vi "DiffDriveSim_FindEncoder.vi"(9 "Restart":bool, 10 "Enc B DI Channel":T1, 11 "Enc A DI Channel":T1) -> (1 "Found":bool, 3 "EncoderIndex":T2)   [LabVIEW 2019]
uses:
  <vilib>/Rock Robotics/SystemInterfaces/Encoder/FPGA_EncoderIdx.ctl
  <vilib>/Rock Robotics/SystemInterfaces/DIO/FPGA_DIOChannel.ctl
  <vilib>/Rock Robotics/WPI/Simulation/Protocol/Devices/Encoder/Encoder Update Ops.ctl
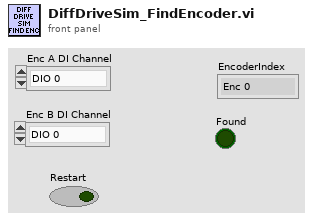
[diagram p1: front panel]
types:
  T1 = typedef "FPGA_DIOChannel.ctl" = enum8{"DIO 0", "DIO 1", "DIO 2", "DIO 3", "DIO 4", "DIO 5", "DIO 6", "DIO 7", "DIO 8", "DIO 9", "DIO MXP 0", "DIO MXP 1", "DIO MXP 2", "DIO MXP 3", "DIO MXP 4", "DIO MXP 5", "DIO MXP 6", "DIO MXP 7", "DIO MXP 8", "DIO MXP 9", "DIO MXP 10", "DIO MXP 11", "DIO MXP 12", "DIO MXP 13", "DIO MXP 14", "DIO MXP 15", "SPI Port CS1", "SPI Port CS2", "SPI Port CS3", "SPI Port MISO", "SPI Port MOSI", "Invalid"}
  T2 = typedef "FPGA_EncoderIdx.ctl" = enum8{"Enc 0", "Enc 1", "Enc 2", "Enc 3", "Enc 4", "Enc 5", "Enc 6", "Enc 7", "Invalid"}
  T3 = typedef "Encoder Update Ops.ctl" = enum16{"set init", "set count", "set period", "set reset", "set samples_to_avg", "get", "delete", "JSON update", "set name", "transmit initial", "reset", "set channel_a", "set channel_b", "set values"}
  T4 = typedef "Encoder proto.ctl" = cluster{"type":string, "device":string, "name":string, "data":T5}
  T5 = typedef "Encoder data protoo.ctl" = cluster{"<init":bool, ">count":dbl, ">period":dbl, "<samples_to_avg":i32, "<offset":dbl, "<channel_a":i32, "<channel_b":i32}
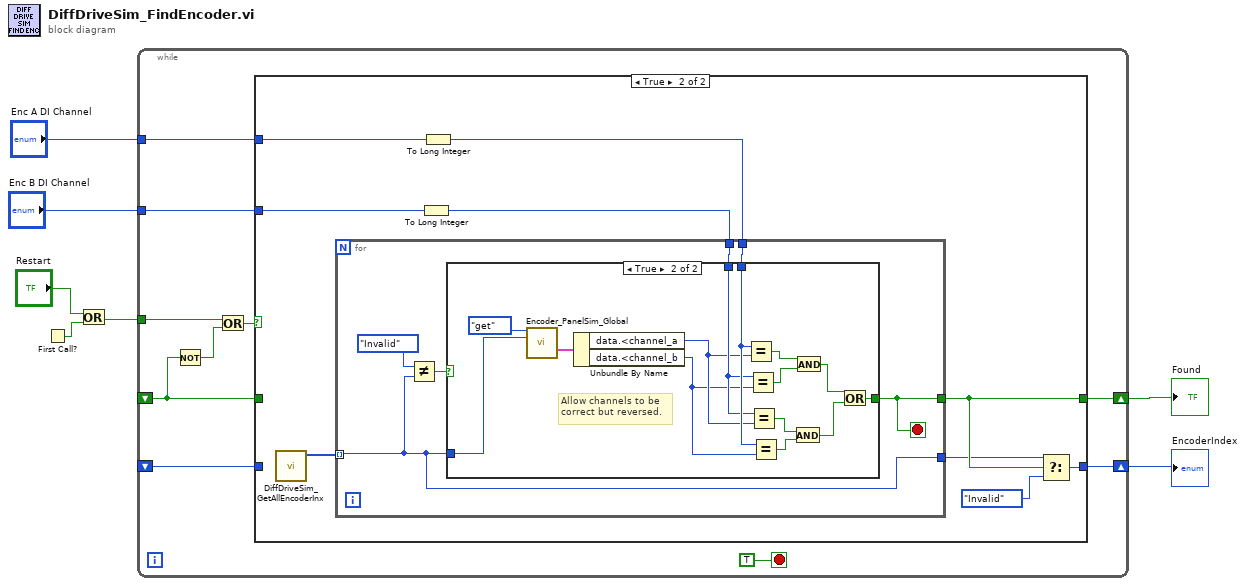
[diagram p0: block diagram]
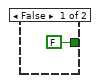
[diagram p3: hidden frame]
diagram:
  n1 = First Call?() -> (First Call?: T/F=w7:bool)
  n2 = Or(x="Restart", y=w7) -> (x .or. y?=w5:bool)
  n3 = while {
    tunnel: w5 -> [w15]
    tunnel: "Enc A DI Channel" -> [w13]
    tunnel: "Enc B DI Channel" -> [w12]
    shift-right: [w11] -> w1
    shift-left: _ -> [w9]
    shift-right: [w10] -> w2
    shift-left: _ -> [w8]
    stop <- TRUE stop-if-true
    n4 = Not(x=w9) -> (.not. x?=w14:bool)
    n5 = Or(x=w15, y=w14) -> (x .or. y?=w16:bool)
    n6 = case shown="True" w16 {
      tunnel: w13 -> [_ w28]
      tunnel: w12 -> [_ w27]
      tunnel: [w19 w24] -> w11
      tunnel: [w18 w22] -> w10
      tunnel: w9 -> [w19 _]
      tunnel: w8 -> [w18 _]
      frame False {
      }
      frame True {
        n7 = call "DiffDriveSim_GetAllEncoderInx.vi"() -> ("All Encoder Inx"=w21:T2[])  [unwired: 11 in]
        n8 = To Long Integer(number=w27) -> (32bit integer=w25:i32)
        n9 = To Long Integer(number=w28) -> (32bit integer=w26:i32)
        n10 = for {
          tunnel: w21 -> [w30] mode=indexing
          tunnel: w26 -> [w34]
          tunnel: w25 -> [w33]
          tunnel: [w32] -> w24
          tunnel: [w30] -> w23
          stop <- w32 stop-if-true
          n11 = Not Equal?(x=FPGA_EncoderIdx."Invalid", y=w30) -> (x != y?=w31:bool)
          n12 = case shown="True" w31 {
            tunnel: w34 -> [_ w47]
            tunnel: w33 -> [_ w46]
            tunnel: [FALSE w37] -> w32
            tunnel: w30 -> [_ w36]
            frame False {
            }
            frame True {
              # "Allow channels to be\ncorrect but reversed."
              n13 = call <vilib>:"Encoder_PanelSim_Global.vi"("menu"=Encoder_Update_Ops."get", "EncoderIndex"=w36) -> ("Encoder new"=w49:T4)  [unwired: 12 in, 1 out]
              n14 = Unbundle By Name(w49) -> ("data.<channel_a"=w45:i32, "data.<channel_b"=w44:i32)
              n15 = Equal?(x=w47, y=w45) -> (x = y?=w42:bool)
              n16 = Equal?(x=w46, y=w44) -> (x = y?=w43:bool)
              n17 = Equal?(x=w46, y=w45) -> (x = y?=w41:bool)
              n18 = Equal?(x=w47, y=w44) -> (x = y?=w40:bool)
              n19 = And(x=w41, y=w40) -> (x .and. y?=w38:bool)
              n20 = And(x=w42, y=w43) -> (x .and. y?=w39:bool)
              n21 = Or(x=w39, y=w38) -> (x .or. y?=w37:bool)
            }
          }
        }
        n22 = Select(t=w23, s=w24, f=FPGA_EncoderIdx."Invalid") -> (s? t:f=w22:T2)
      }
    }
  }
  "EncoderIndex" <- w2
  "Found" <- w1
